vi "ReceiveStreamData.vi"(8 "Error In":errorcluster, 9 "Timeout (ms)":i32, 11 "Connection In":T4={"UDP Connection ID"=refnum, "TCP Connection ID"=refnum, "Remote UDP Port"=61557, "Remote IP"=0}) -> (0 "Error Out":errorcluster, 2 "ClientStreamData":T1, 3 "Connection Out":T4={"UDP Connection ID"=refnum, "TCP Connection ID"=refnum, "Remote UDP Port"=61557, "Remote IP"=0}, 4 "stop?":bool)   [LabVIEW 2017, in "Game.lvlib" / "GameComms.lvlib"]
uses:
  GameComms.lvlib
  TypeDefs/Connection.ctl
  TypeDefs/ClientStreamData.ctl
  TypeDefs/TargetPosition.ctl
  TypeDefs/ForceVector.ctl
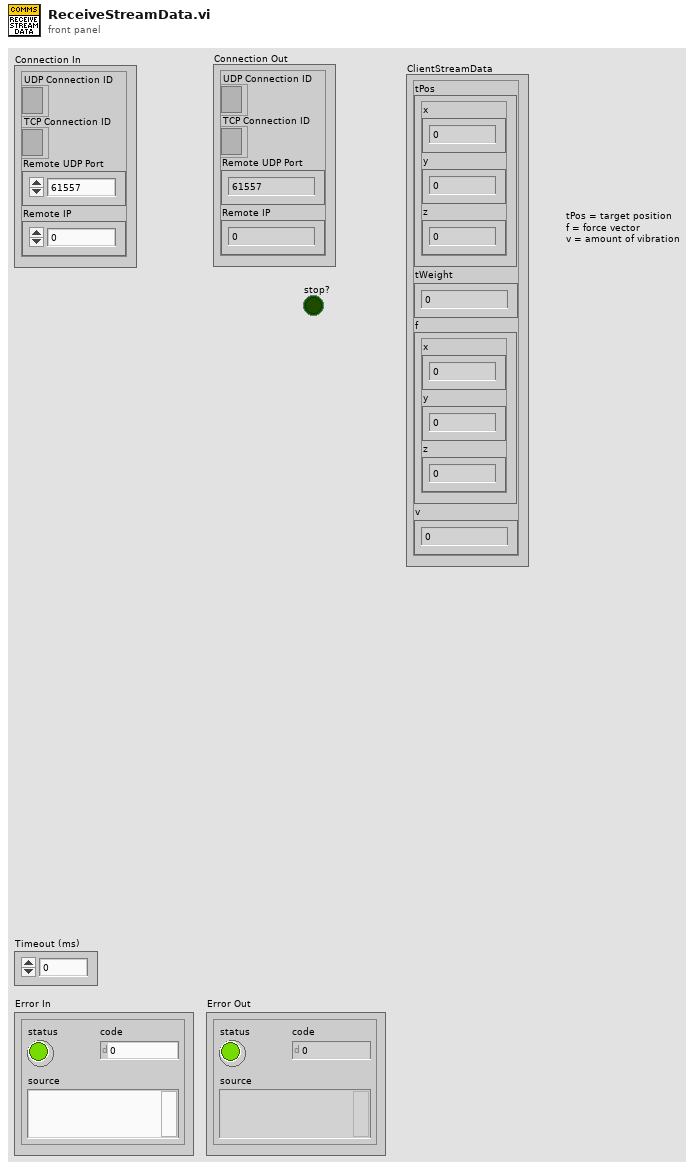
[diagram p1: front panel]
types:
  T1 = typedef "Game.lvlib/GameComms.lvlib/ClientStreamData.ctl" = cluster{"tPos":T2, "tWeight":dbl, "f":T3, "v":dbl}
  T2 = typedef "Game.lvlib/GameComms.lvlib/TargetPosition.ctl" = cluster{"x":dbl, "y":dbl, "z":dbl}
  T3 = typedef "Game.lvlib/GameComms.lvlib/ForceVector.ctl" = cluster{"x":dbl, "y":dbl, "z":dbl}
  T4 = typedef "Game.lvlib/GameComms.lvlib/Connection.ctl" = cluster{"UDP Connection ID":refnum<k16>, "TCP Connection ID":refnum<k5>, "Remote UDP Port":u16, "Remote IP":u32}
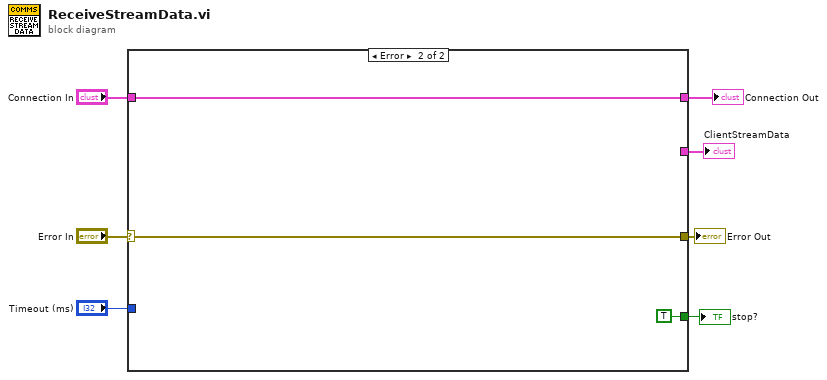
[diagram p0: block diagram]
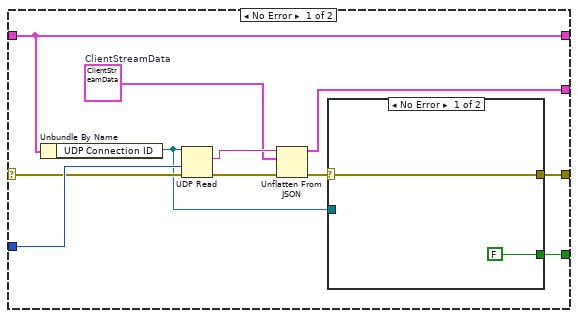
[diagram p2: hidden frame]
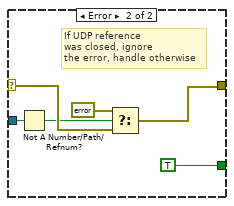
[diagram p3: hidden frame]
diagram:
  n1 = case shown="Error" "Error In" {
    selector: "Error In" -> [w14 w29]
    tunnel: [w10 w29] -> w6
    tunnel: "Connection In" -> [w13 w28]
    tunnel: [w13 w28] -> w4
    tunnel: "Timeout (ms)" -> [w15 _]
    tunnel: [w16 _] -> w2
    tunnel: [w9 TRUE] -> w1
    frame No Error {
      w17 = T1 {"tPos"={"x"=0.0, "y"=0.0, "z"=0.0}, "tWeight"=0.0, "f"={"x"=0.0, "y"=0.0, "z"=0.0}, "v"=0.0}  # ClientStreamData
      n2 = Unbundle By Name(w13) -> ("UDP Connection ID"=w8:refnum<k16>)
      n3 = UDP Read(connection ID=w8, timeout ms (25000)=w15, 8:w14) -> (data out=w18:string, error out=w12:errorcluster)  [unwired: 1 in, 3 out]
      n4 = Unflatten From JSON(JSON string=w18, type and defaults=w17, error in (no error)=w12) -> (value=w16:T1, error out=w11:errorcluster)  [unwired: 4 in]
      n5 = case shown="No Error" w11 {
        selector: w11 -> [w20 w26]
        tunnel: [w20 w24] -> w10
        tunnel: [FALSE TRUE] -> w9
        tunnel: w8 -> [_ w21]
        frame No Error {
        }
        frame Error {
          # "If UDP reference\nwas closed, ignore\nthe error, handle otherwise"
          n6 = Not A Number/Path/Refnum?(number/path/refnum=w21) -> (NaN/Path/Refnum?=w22:bool)
          n7 = Select(t=errorcluster {"status"=FALSE, "code"=0, "source"=""}, s=w22, f=w26) -> (s? t:f=w24:errorcluster)
        }
      }
    }
    frame Error {
    }
  }
  "Error Out" <- w6
  "Connection Out" <- w4
  "ClientStreamData" <- w2
  "stop?" <- w1
